vi "Size Grove.vi"(10 "Elf Locations":T1[](array[typedef]), 11 "Original Grove":T2[][](array[typedef])) -> (2 "Elf Locations 2":T1[](array[typedef]), 3 "Spaced Grove":T2[][](array[typedef]))   [LabVIEW 2020]
uses:
  Cluster _Point Location.ctl
  RB ENUM_Spot ID.ctl
  78f477a4-3fa2-46a3-afd1-ccb2ea7daf80.vi
  6a400570-d694-4cff-9be2-ef43f19114a4.vi
  903fd045-1e6e-4ac9-b45e-ec3af8625212.vi
  3d876b91-80d9-4741-b626-61ba73055adf.vi
  <vilib>/Comparison/Equal/Equal Functor/Equal Functor.lvclass
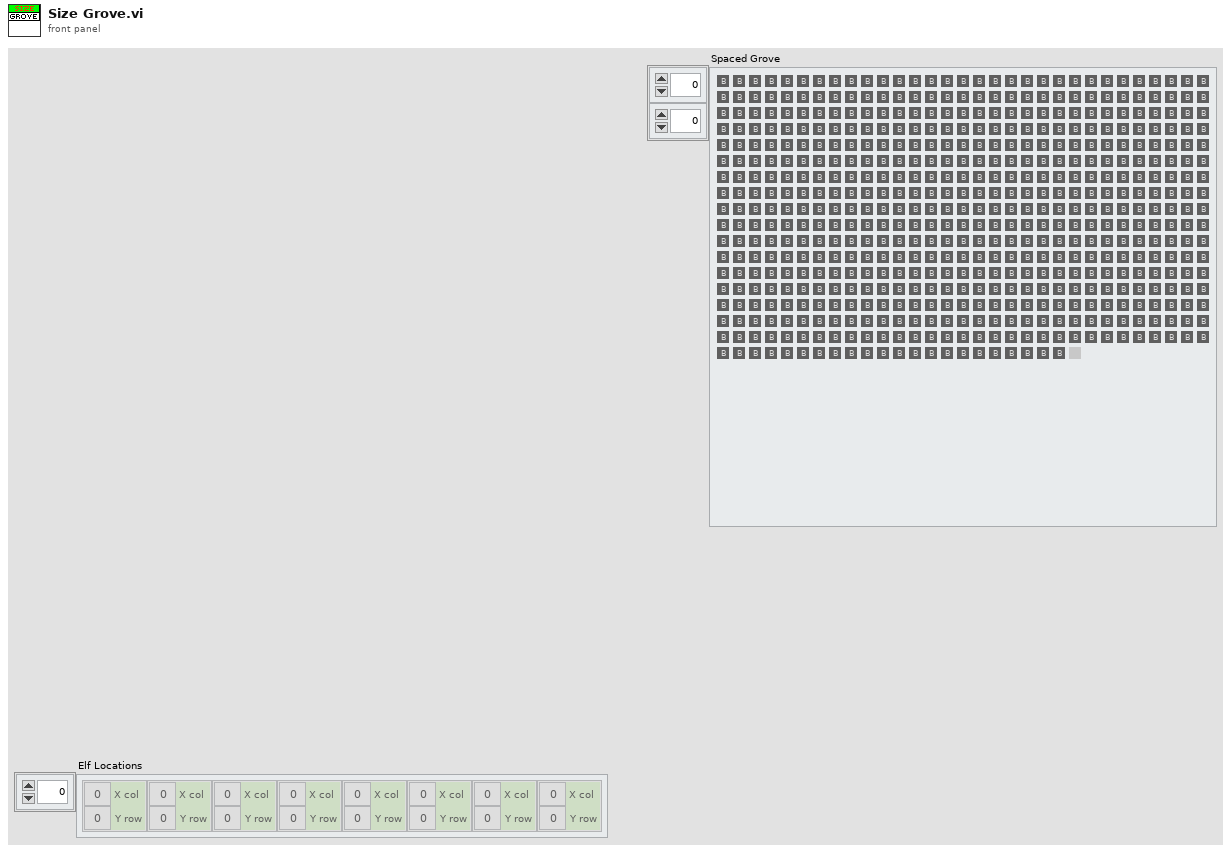
[diagram p1: front panel]
types:
  T1 = typedef "Cluster _Point Location.ctl" = cluster{"X col":i32, "Y row":i32}
  T2 = typedef "RB ENUM_Spot ID.ctl" = enum32{"Blank", "ELF", "Proposed"}
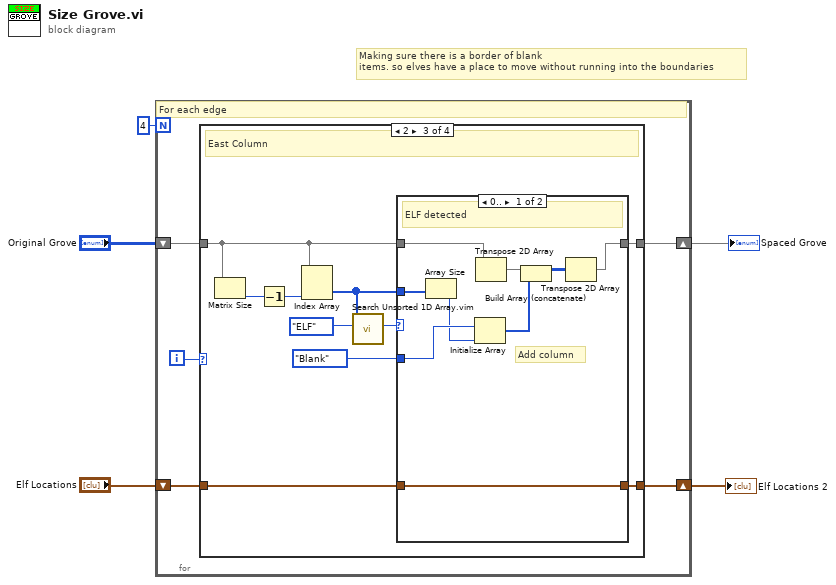
[diagram p0: block diagram]
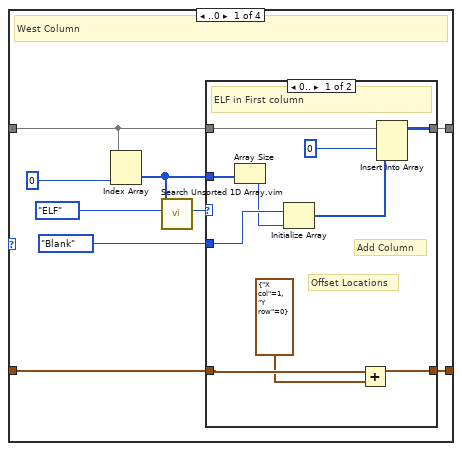
[diagram p2: hidden frame]
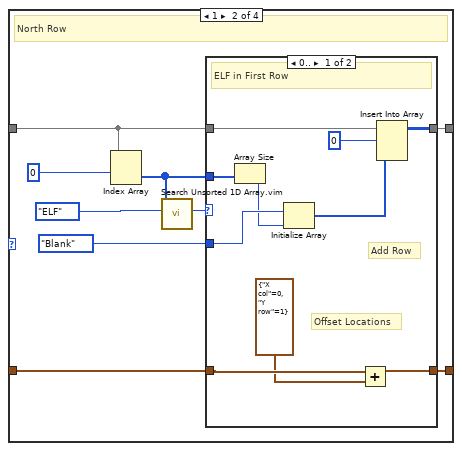
[diagram p4: hidden frame]
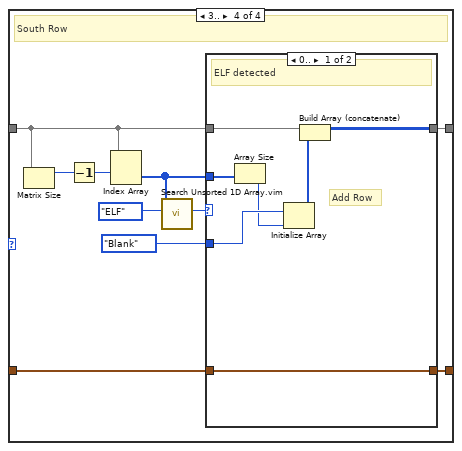
[diagram p7: hidden frame]
diagram:
  # "Making sure there is a border of blank\nitems. so elves have a place to move without running into the boundaries"
  n1 = for {
    N: 4 -> [_]
    shift-right: [w8] -> w4
    shift-left: "Original Grove" -> [w9]
    shift-right: [w6] -> w2
    shift-left: "Elf Locations" -> [w7]
    i -> [w10]
    # "For each edge"
    n2 = case shown="2" w10 {
      tunnel: w9 -> [w16 w38 w55 w76]
      tunnel: [w15 w37 w60 w81] -> w8
      tunnel: w7 -> [w14 w36 w59 w80]
      tunnel: [w13 w35 w58 w79] -> w6
      frame ..0 {
        # "West Column"
        n3 = Index Array(array=w16, index (col)=0 ("disabled index (col)")) -> (element=w12:T2[])  [unwired: 1 in]
        n4 = call "Search Unsorted 1D Array.vim"("element"=RB_ENUM_Spot_ID."ELF" ("Spot"), "unsorted 1D array"=w12) -> ("index of element"=w17:i32)  [unwired: 9 in]
        n5 = case shown="0.." w17 {
          tunnel: w16 -> [w26 w31]
          tunnel: [w25 w31] -> w15
          tunnel: w14 -> [w22 w30]
          tunnel: [w21 w30] -> w13
          tunnel: w12 -> [w29 _]
          tunnel: RB_ENUM_Spot_ID."Blank" ("Spot") -> [w28 _]
          frame 0.. {
            # "Offset Locations"
            # "Add Column"
            # "ELF in First column"
            n6 = Array Size(array=w29) -> (size(s)=w27:i32)
            n7 = Initialize Array(w28, w27) -> (w23:T2[])
            n8 = Add(x=w22, y=T1 {"X col"=1, "Y row"=0} ("Point")) -> (x+y=w21:T1[])
            n9 = Insert Into Array(array=w26, index (col)=0 ("disabled index (col)"), new element=w23) -> (w25:T2[][])  [unwired: 1 in]
          }
          frame ..-1 {
            # "No Elf Detected"
          }
        }
      }
      frame 1 {
        # "North Row"
        n10 = Index Array(array=w38, index (row)=0 ("disabled index (col)")) -> (element=w34:T2[])  [unwired: 1 in]
        n11 = call "Search Unsorted 1D Array.vim"("element"=RB_ENUM_Spot_ID."ELF" ("Spot"), "unsorted 1D array"=w34) -> ("index of element"=w39:i32)  [unwired: 9 in]
        n12 = case shown="0.." w39 {
          tunnel: w38 -> [w47 w52]
          tunnel: [w46 w52] -> w37
          tunnel: w36 -> [w44 w51]
          tunnel: [w43 w51] -> w35
          tunnel: w34 -> [w50 _]
          tunnel: RB_ENUM_Spot_ID."Blank" ("Spot") -> [w49 _]
          frame 0.. {
            # "Offset Locations"
            # "Add Row"
            # "ELF in First Row"
            n13 = Array Size(array=w50) -> (size(s)=w48:i32)
            n14 = Initialize Array(w49, w48) -> (w45:T2[])
            n15 = Add(x=w44, y=T1 {"X col"=0, "Y row"=1} ("Point")) -> (x+y=w43:T1[])
            n16 = Insert Into Array(array=w47, index (row)=0 ("disabled index (col)"), new element=w45) -> (w46:T2[][])  [unwired: 1 in]
          }
          frame ..-1 {
            # "No Elf Detected"
          }
        }
      }
      frame 2 {
        # "East Column"
        n17 = Matrix Size(0:w55) -> (2:w53:i32)  [unwired: 1 out]
        n18 = Decrement(x=w53) -> (x-1=w54:i32)
        n19 = Index Array(array=w55, index (col)=w54) -> (element=w57:T2[])  [unwired: 1 in]
        n20 = call "Search Unsorted 1D Array.vim"("element"=RB_ENUM_Spot_ID."ELF" ("Spot"), "unsorted 1D array"=w57) -> ("index of element"=w61:i32)  [unwired: 9 in]
        n21 = case shown="0.." w61 {
          tunnel: w55 -> [w66 w73]
          tunnel: [w67 w73] -> w60
          tunnel: w59 -> [w68 w72]
          tunnel: [w68 w72] -> w58
          tunnel: w57 -> [w71 _]
          tunnel: RB_ENUM_Spot_ID."Blank" ("Spot") -> [w70 _]
          frame 0.. {
            # "Add column"
            # "ELF detected"
            n22 = Array Size(array=w71) -> (size(s)=w69:i32)
            n23 = Initialize Array(w70, w69) -> (w63:T2[])
            n24 = Transpose 2D Array(2D array=w66) -> (transposed array=w65:T2[][])
            n25 = Build Array (concatenate)(w65, w63) -> (w64:T2[][])
            n26 = Transpose 2D Array(2D array=w64) -> (transposed array=w67:T2[][])
          }
          frame ..-1 {
            # "No Elf Detected"
          }
        }
      }
      frame 3.. {
        # "South Row"
        n27 = Matrix Size(0:w76) -> (1:w74:i32)  [unwired: 1 out]
        n28 = Decrement(x=w74) -> (x-1=w75:i32)
        n29 = Index Array(array=w76, index (row)=w75) -> (element=w78:T2[])  [unwired: 1 in]
        n30 = call "Search Unsorted 1D Array.vim"("element"=RB_ENUM_Spot_ID."ELF" ("Spot"), "unsorted 1D array"=w78) -> ("index of element"=w82:i32)  [unwired: 9 in]
        n31 = case shown="0.." w82 {
          tunnel: w76 -> [w85 w92]
          tunnel: [w84 w92] -> w81
          tunnel: w80 -> [w87 w91]
          tunnel: [w87 w91] -> w79
          tunnel: w78 -> [w90 _]
          tunnel: RB_ENUM_Spot_ID."Blank" ("Spot") -> [w89 _]
          frame 0.. {
            # "Add Row"
            # "ELF detected"
            n32 = Array Size(array=w90) -> (size(s)=w88:i32)
            n33 = Initialize Array(w89, w88) -> (w86:T2[])
            n34 = Build Array (concatenate)(w85, w86) -> (w84:T2[][])
          }
          frame ..-1 {
            # "No Elf Detected"
          }
        }
      }
    }
  }
  "Spaced Grove" <- w4
  "Elf Locations 2" <- w2
